vi "SetArmPosition.vi"(1 "ArmYPosition":dbl, 2 "ArmXPosition":dbl) -> ()   [LabVIEW 2017]
uses:
  <vilib>/Rock Robotics/Network Tables/NT Write Number.vi
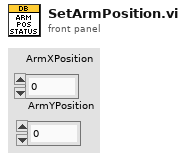
[diagram p1: front panel]
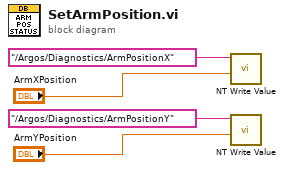
[diagram p0: block diagram]
diagram:
  n1 = call-poly <vilib>:"NT Write Value.vi"("Numeric"="ArmXPosition", "Name"="/Argos/Diagnostics/ArmPositionX") -> ()  [unwired: 9 in, 1 out]
  n2 = call-poly <vilib>:"NT Write Value.vi"("Numeric"="ArmYPosition", "Name"="/Argos/Diagnostics/ArmPositionY") -> ()  [unwired: 9 in, 1 out]
